vi "ModPha2ReIm.vi"(10 "Phase":dbl format="%.6e", 11 "Module dB":dbl format="%.6e") -> (0 "Inv_Im":dbl format="%.6e", 1 "Inv_Re":dbl format="%.6e", 2 "Imag":dbl format="%.6e", 3 "Real":dbl format="%.6e")   [LabVIEW 2017]
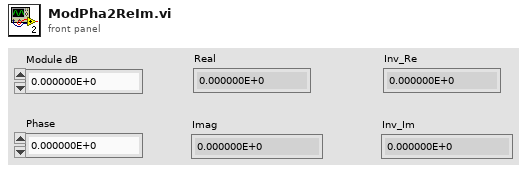
[diagram p1: front panel]
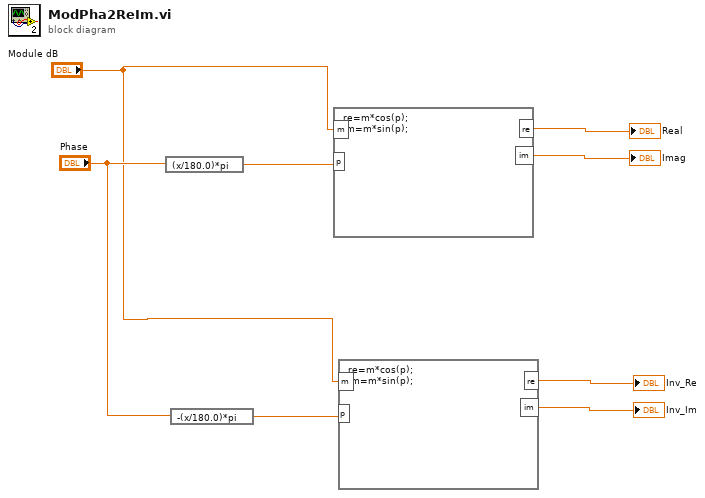
[diagram p0: block diagram]
diagram:
  n1 = expression code="(x/180.0)*pi" ("degrees to radians")("Phase") -> (w6:dbl)
  n2 = expression code="-(x/180.0)*pi" ("degrees to radians")("Phase") -> (w5:dbl)
  n3 = formula code="re=m*cos(p);\nim=m*sin(p);"("m"="Module dB", "p"=w6) -> ("re"=→"Real":dbl, "im"=→"Imag":dbl)
  n4 = formula code="re=m*cos(p);\nim=m*sin(p);"("m"="Module dB", "p"=w5) -> ("re"=→"Inv_Re":dbl, "im"=→"Inv_Im":dbl)
